vi "Op-Start-Stop.vi"(6 "time to wait (30000ms)":i32=30000, 8 "error in (no error)":errorcluster, 9 "function (stop:0)":i32(slide) scale=0.0..7.0, 10 "wait until finish":bool=TRUE, 11 "VISA resource name":refnum<visa-resource-name>) -> (0 "error out":errorcluster, 3 "VISA resource name out":refnum<visa-resource-name>)   [LabVIEW 2016, in "Agilent 415X Series.lvlib"]
doc: "This VI controls the instrument's execution state by starting or stopping a sweep/sampling measurement or stress mode opeation.\n\nIf synchronous execution is desired when performing a measurement or a stress test, set \"Wait Until Finish\" control to YES, which uses the instrument's Opeartion Complete Status Bits to monitor the exection status and causes the VI to return only when the measurement/stress operation is finished.\n\n*Notice: when doing an asynchronous execution, the default timeout \n value is set at 60000 ms or 1 min. However, if there is any \n measurement that requires to run more than 50 seconds, \n the user needs to raise the timeout value to accommodate the setup."
uses:
  Agilent 415X Series.lvlib
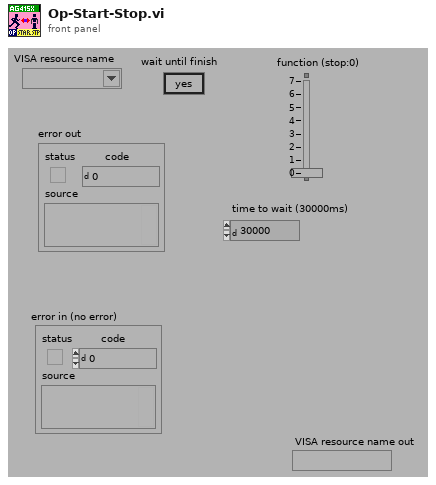
[diagram p1: front panel]
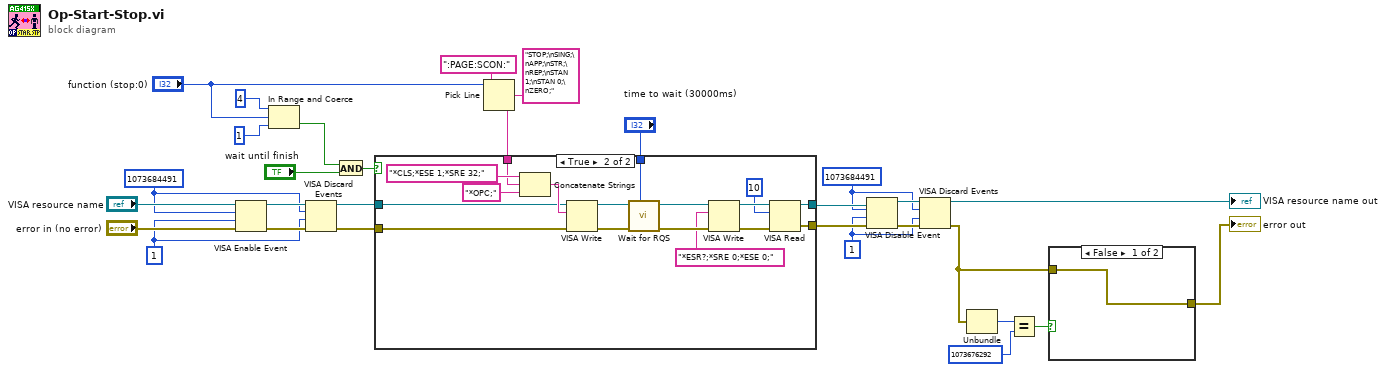
[diagram p0: block diagram]
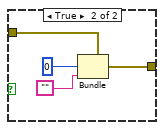
[diagram p2: hidden frame]
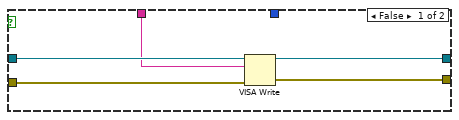
[diagram p3: hidden frame]
diagram:
  w13 = u16 1
  w14 = u32 1073684491
  w9 = u16 1
  w10 = u32 1073684491
  n1 = VISA Enable Event(8:"error in (no error)", 9:w9, 10:w10, 11:"VISA resource name") -> (0:w11:errorcluster, 3:w12:refnum<visa-resource-name>)
  n2 = In Range and Coerce(upper limit=4, x="function (stop:0)", lower limit=1) -> (In Range?=w26:bool)  [unwired: 1 out]
  n3 = VISA Discard Events(8:w11, 9:w9, 10:w10, 11:w12) -> (0:w7:errorcluster, 3:w8:refnum<visa-resource-name>)
  n4 = And(x=w26, y="wait until finish") -> (x .and. y?=w23:bool)
  n5 = Pick Line(string ("")=":PAGE:SCON:", multi-line string="STOP;\nSING;\nAPP;\nSTR;\nREP;\nSTAN 1;\nSTAN 0;\nZERO;", line index="function (stop:0)") -> (output string=w21:string)
  n6 = case shown="True" w23 {
    tunnel: [w34 w45] -> w17
    tunnel: "time to wait (30000ms)" -> [_ w50]
    tunnel: w21 -> [w33 w46]
    tunnel: w8 -> [w35 w38]
    tunnel: [w32 w37] -> w18
    tunnel: w7 -> [w31 w36]
    frame False {
      n7 = VISA Write(VISA resource name=w35, write buffer=w33, error in (no error)=w31) -> (VISA resource name out=w32:refnum<visa-resource-name>, error out=w34:errorcluster)  [unwired: 1 out]
    }
    frame True {
      n8 = Concatenate Strings("*CLS;*ESE 1;*SRE 32;", w46, "*OPC;") -> (w48:string)
      n9 = VISA Write(VISA resource name=w38, write buffer=w48, error in (no error)=w36) -> (VISA resource name out=w51:refnum<visa-resource-name>, error out=w52:errorcluster)  [unwired: 1 out]
      n10 = call <vilib>:"Wait for RQS.VI"("timeout (25000 ms)"=w50, "error in (no error)"=w52, "VISA resource name"=w51) -> ("error out"=w43:errorcluster, "VISA resource name out"=w42:refnum<visa-resource-name>)  [unwired: 6 in, 1 out]
      n11 = VISA Write(VISA resource name=w42, write buffer="*ESR?;*SRE 0;*ESE 0;", error in (no error)=w43) -> (VISA resource name out=w41:refnum<visa-resource-name>, error out=w44:errorcluster)  [unwired: 1 out]
      n12 = VISA Read(VISA resource name=w41, byte count=u32 10, error in (no error)=w44) -> (VISA resource name out=w37:refnum<visa-resource-name>, error out=w45:errorcluster)  [unwired: 2 out]
    }
  }
  n13 = VISA Disable Event(8:w17, 9:w13, 10:w14, 11:w18) -> (0:w15:errorcluster, 3:w16:refnum<visa-resource-name>)
  n14 = VISA Discard Events(8:w15, 9:w13, 10:w14, 11:w16) -> (0:w3:errorcluster, 3:→"VISA resource name out":refnum<visa-resource-name>)
  n15 = Unbundle(w3) -> ("code"=w6:i32)  [unwired: 2 out]
  n16 = Equal?(x=w6, y=1073676292) -> (x = y?=w4:bool)
  n17 = case shown="False" w4 {
    tunnel: w3 -> [w53 w57]
    tunnel: [w53 w56] -> w2
    frame False {
    }
    frame True {
      n18 = Bundle(cluster=w57, "code"=0, "source"="") -> (w56:errorcluster)  [unwired: 1 in]
    }
  }
  "error out" <- w2
